vi "Run Self-Calibration.vi"(8 "error in (no error)":errorcluster, 11 "VISA resource name":refnum<visa-resource-name>) -> (0 "error out":errorcluster, 2 "Calibration Successful":bool, 3 "VISA resource name out":refnum<visa-resource-name>)   [LabVIEW 2017, in "RadWag balances and scales.lvlib"]
doc: "Runs internal calibration of balance."
uses:
  <instrlib>/Radwag Balances and Scales/Public/RadWag balances and scales.lvlib
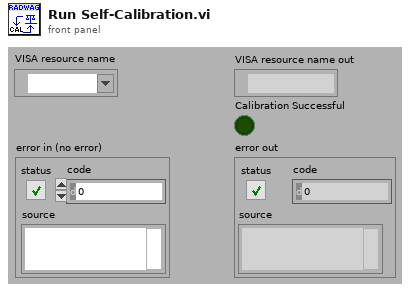
[diagram p1: front panel]
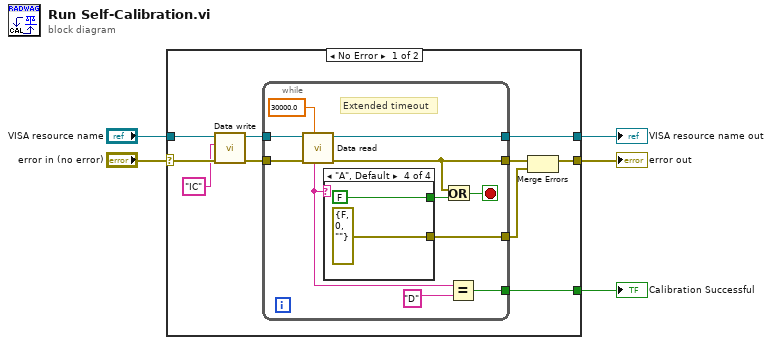
[diagram p0: block diagram]
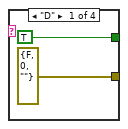
[diagram p2: hidden frame]
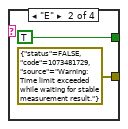
[diagram p3: hidden frame]
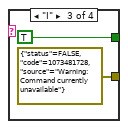
[diagram p4: hidden frame]
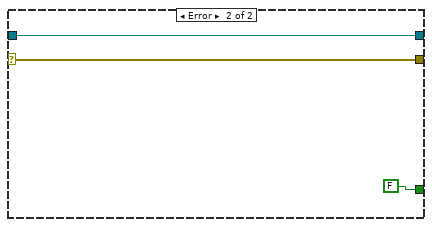
[diagram p5: hidden frame]
diagram:
  n1 = case shown="No Error" "error in (no error)" {
    selector: "error in (no error)" -> [w11 w36]
    tunnel: "VISA resource name" -> [w15 w37]
    tunnel: [w12 w37] -> w4
    tunnel: [w8 w36] -> w3
    tunnel: [w6 FALSE] -> w1
    frame No Error {
      n2 = call <instrlib>:"Data write.vi"("error in (no error)"=w11, "ID"="IC", "VISA resource name"=w15) -> ("error out"=w13:errorcluster, "VISA resource name out"=w14:refnum<visa-resource-name>)  [unwired: 7 in]
      n3 = while {
        tunnel: w14 -> [w26]
        tunnel: w13 -> [w25]
        tunnel: [w24] -> w12
        tunnel: [w21] -> w9
        tunnel: [w19] -> w7
        tunnel: [w16] -> w6
        stop <- w23 stop-if-true
        # "Extended timeout"
        n4 = call <instrlib>:"Data read.vi"("Timeout [ms]"=30000.0, "error in (no error)"=w25, "VISA resource name"=w26) -> ("error out"=w21:errorcluster, "VISA resource name out"=w24:refnum<visa-resource-name>, "Status"=w18:string)  [unwired: 2 in, 4 out]
        n5 = case shown="\"A\", Default" w18 {
          tunnel: [TRUE TRUE TRUE FALSE] -> w20
          tunnel: [errorcluster {"status"=FALSE, "code"=0, "source"=""} ("error constant") errorcluster {"status"=FALSE, "code"=1073481729, "source"="Warning: Time limit exceeded while waiting for stable measurement result."} ("t") errorcluster {"status"=FALSE, "code"=1073481728, "source"="Warning: Command currently unavailable"} ("t") errorcluster {"status"=FALSE, "code"=0, "source"=""} ("error constant")] -> w19
          frame "D" {
          }
          frame "E" {
          }
          frame "I" {
          }
          frame "A", Default {
          }
        }
        n6 = Or(x=w21, y=w20) -> (x .or. y?=w23:bool)
        n7 = Equal?(x=w18, y="D") -> (x = y?=w16:bool)
      }
      n8 = Merge Errors(w9, w7) -> (w8:errorcluster)
    }
    frame Error {
    }
  }
  "error out" <- w3
  "VISA resource name out" <- w4
  "Calibration Successful" <- w1
